vi "Test_DS3.vi"() -> ()   [LabVIEW 2015]
uses:
  controls/PS3 Controls.ctl
  <vilib>/Utility/inputDevices.llb/closeJoystick.vi
panel:
  out "u8":u8[](array[numeric])
  out "uint 8":u8[](array[numeric])
  out "int32":i32[](array[numeric])
  out "error out":errorcluster
  in  "stop":bool
  out "PS3 Controls":T1 {"Left Analogue Stick X" scale=-32768.0..32768.0; "Left Analogue Stick Y" scale=32768.0..-32768.0; "Right Analogue Stick X" scale=-32768.0..32768.0; "Right Analogue Stick Y" scale=32768.0..-32768.0; "X Rotation" scale=-32768.0..32768.0; "Y Rotation" scale=-32768.0..32768.0; "L2 Pressure" scale=0.0..32768.0; "Numeric" format="%d°"}
  # "Left X"
  # "Left Y"
  # "Right X"
  # "Right Y"
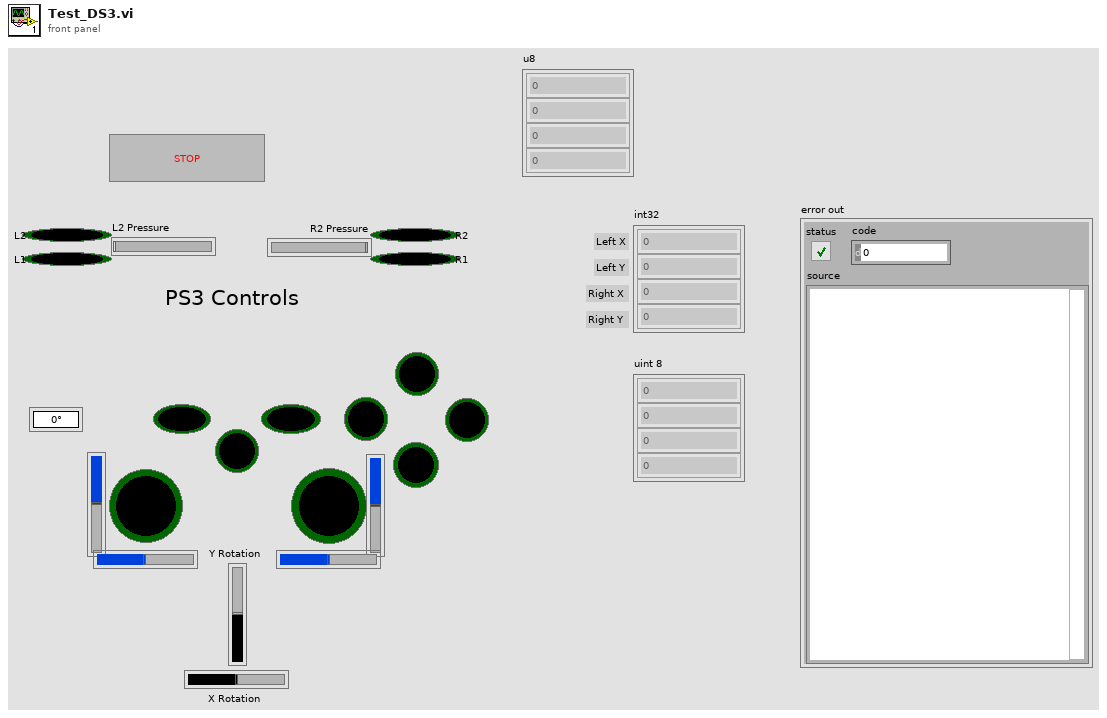
[diagram p1: front panel]
types:
  T1 = typedef "PS3 Controls.ctl" = cluster{"Left Analogue Stick X":i32, "Left Analogue Stick Y":i32, "Right Analogue Stick X":i32, "Right Analogue Stick Y":i32, "Y Rotation":i32, "X Rotation":i32, "L2 Pressure":i32, "R2 Pressure":i32, "Triangle":bool, "Circle":bool, "X":bool, "Square":bool, "L1":bool, "R1":bool, "L2":bool, "R2":bool, "L3":bool, "R3":bool, "Select":bool, "Start":bool, "PS Button":bool, "Numeric":i32}
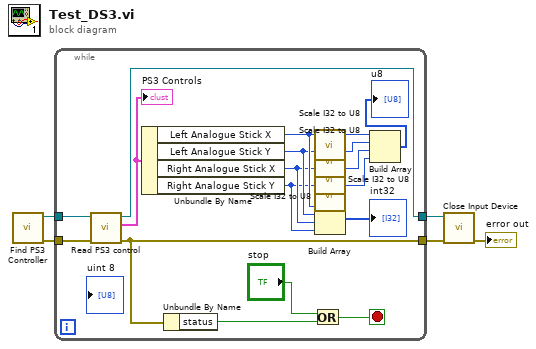
[diagram p0: block diagram]
diagram:
  n1 = call "Find PS3 Controller.vi"() -> ("error out"=w2:errorcluster, "Controller Reference Out"=w5:refnum<k1>)  [unwired: 10 in]
  n2 = while {
    tunnel: w5 -> [w21]
    tunnel: w2 -> [w22]
    tunnel: [w23] -> w4
    tunnel: [w18] -> w3
    stop <- w19 stop-if-true
    n3 = call "Read PS3 control.vi"("error in (no error)"=w22, "Controller Reference In"=w21) -> ("error out"=w18:errorcluster, "PS3 Controls"=w16:T1, "Controller Reference Out"=w23:refnum<k1>)  [unwired: 7 in]
    "PS3 Controls" <- w16
    n4 = Unbundle By Name(w16) -> ("Left Analogue Stick X"=w10:i32, "Left Analogue Stick Y"=w9:i32, "Right Analogue Stick X"=w8:i32, "Right Analogue Stick Y"=w7:i32)
    n5 = Unbundle By Name(w18) -> ("status"=w17:bool)
    n6 = Or(x="stop", y=w17) -> (x .or. y?=w19:bool)
    n7 = call "Scale I32 to U8.vi"("Input"=w10) -> ("Output"=w14:u8)  [unwired: 4 in]
    n8 = call "Scale I32 to U8.vi"("Input"=w9) -> ("Output"=w13:u8)  [unwired: 4 in]
    n9 = call "Scale I32 to U8.vi"("Input"=w8) -> ("Output"=w12:u8)  [unwired: 4 in]
    n10 = call "Scale I32 to U8.vi"("Input"=w7) -> ("Output"=w11:u8)  [unwired: 4 in]
    n11 = Build Array(w10, w9, w8, w7) -> (→"int32":i32[])
    n12 = Build Array(w14, w13, w12, w11) -> (→"u8":u8[])
  }
  n13 = call-poly <vilib>:"Close Input Device.vi"("error in (no error)"=w3, "device ID"=w4) -> ("error out"=→"error out":errorcluster)  [unwired: 8 in]
